vi "save_image_acquisition_time_to_textfile.vi"(9 "Input \nparameters":T2={"Frame rate (ms)"=2000, "Worm strain"="N2", "# Images"=0, "State"=enum."Image acquisition", "Acquisition Time"=0.0, "Max_num_runs"=100000, "#TTL"=0, "Time of start TTL"=100000, "ImSub Value"=0, "Time of last TTL"=0, "Number of Columns"=2, "Number of Rows"=2, "# AdjacentTTL"=0, "Sleep deprivation status"="", "Sleep Detection"=FALSE, "# Sleep detections"=0, "Time of first sleep detection"=0, "Time max # adjacent TTL"=0, "Image t-1"=[], "Image t"=[]} {"Number of Rows" items=["1"=1, "2"=2, "3"=3, "4"=4]; "Number of Columns" items=["1"=1, "2"=2, "3"=3, "4"=4]}) -> ()   [LabVIEW 2011]
uses:
  state.ctl
  Action-Init-Update-Get.ctl
  <vilib>/Utility/file.llb/Write To Spreadsheet File (DBL).vi
panel:
  out "Filestem":string
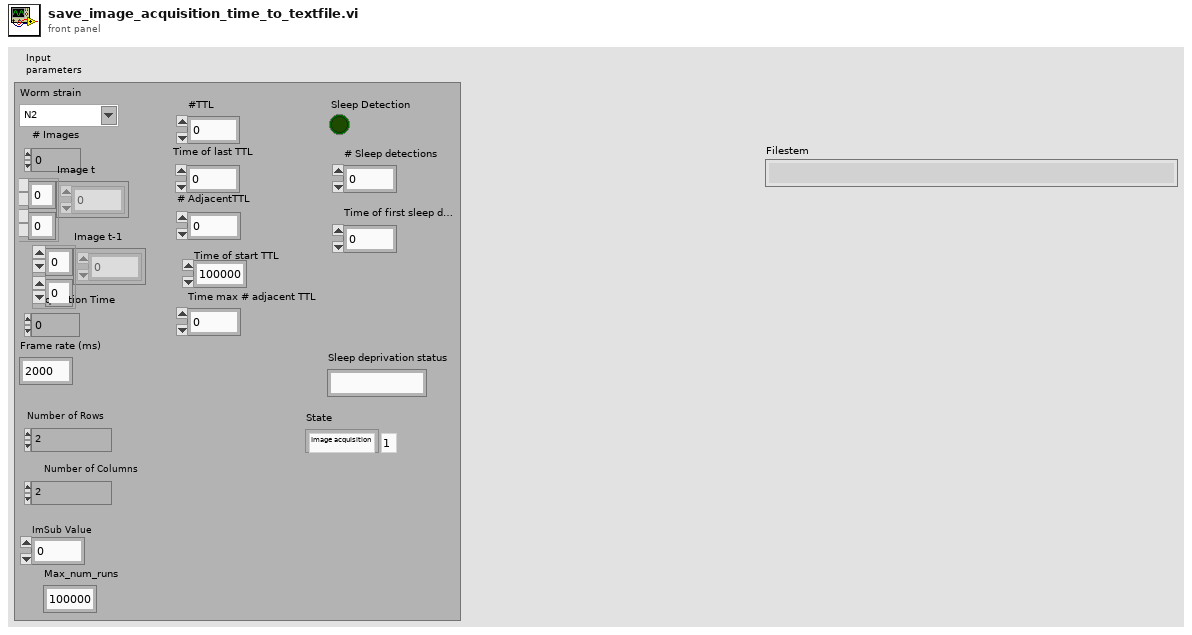
[diagram p1: front panel]
types:
  T1 = typedef "state.ctl" = enum16{"Initialize measurement", "Image acquisition", "Image processing", "Sleep detection", "Control TTL protocol ", "Sleep deprivation", "Update image & exit condition", "Wait "}
  T2 = cluster{"Frame rate (ms)":u32, "Worm strain":string, "# Images":i32, "State":T1, "Acquisition Time":dbl, "Max_num_runs":i32, "#TTL":i32, "Time of start TTL":i32, "ImSub Value":i32, "Time of last TTL":i32, "Number of Columns":u32, "Number of Rows":u32, "# AdjacentTTL":i32, "Sleep deprivation status":string, "Sleep Detection":bool, "# Sleep detections":i32, "Time of first sleep detection":i32, "Time max # adjacent TTL":i32, "Image t-1":i32[][], "Image t":i32[][]}
  T3 = typedef "Action-Init-Update-Get.ctl" = enum16{"Initialize", "Update", "Get"}
  T4 = cluster{"Path":string, "Filestem":string, "Filestem incl time t":string, "Date":string}
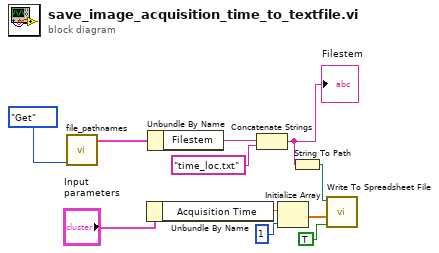
[diagram p0: block diagram]
diagram:
  n1 = call "file_pathnames.vi"("Action"=Action-Init-Update-Get."Get") -> ("File-path\n-names"=w6:T4)  [unwired: 10 in]
  n2 = Unbundle By Name("Input \nparameters") -> ("Acquisition Time"=w4:dbl)
  n3 = Unbundle By Name(w6) -> ("Filestem"=w3:string)
  n4 = Concatenate Strings(w3, "time_loc.txt" ("new file path (Not A Path if cancelled)")) -> (w2:string)
  "Filestem" <- w2
  n5 = Initialize Array(w4, 1 ("Dimension")) -> (w10:dbl[])
  n6 = String To Path(string=w2) -> (path=w8:path)
  n7 = call-poly <vilib>:"Write To Spreadsheet File.vi"("append to file? (new file:F)"=TRUE, "1D data"=w10, "file path (dialog if empty)"=w8) -> ()  [unwired: 5 in, 1 out]
